vi "Request Data JSON.vi"(8 "error in (no error)":errorcluster, 11 "GetInputSettings in":refnum<class "GetInputSettings.lvclass">) -> (0 "error out":errorcluster, 2 "Request Data JSON":string, 3 "GetInputSettings out":refnum<class "GetInputSettings.lvclass">)   [LabVIEW 2022 SP3, in "obs-websocket-lv.lvlib" / "GetInputSettings.lvclass"]
uses:
  GetInputSettings.lvclass
  GetInputSettings.lvclass/GetInputSettings.ctl
  <vilib>/IlluminatedG/lv-web-crypto/lv-json/JSON/JSON.lvlib
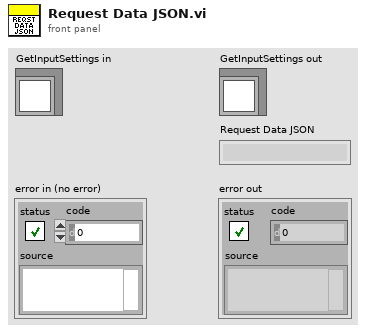
[diagram p1: front panel]
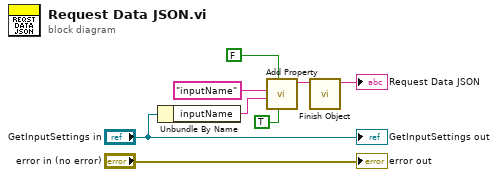
[diagram p0: block diagram]
diagram:
  n1 = Unbundle By Name("GetInputSettings in") -> ("inputName"=w5:string)
  n2 = call <vilib>:"Add Property.vi"("String?"=TRUE, "Include Empty?"=FALSE, "Value"=w5, "Property Name"="inputName") -> ("String out"=w3:string)  [unwired: 7 in]
  n3 = call <vilib>:"Finish Object.vi"("String In"=w3) -> ("String out"=→"Request Data JSON":string)  [unwired: 10 in]
  "error out" <- "error in (no error)"
  "GetInputSettings out" <- "GetInputSettings in"
